vi "Type Conversion.To Double (I8).vi"(3 "value in":i8) -> (1 "value out":dbl)   [LabVIEW 2016, in "VeriStand Data.lvlib"]
doc: "Converts the provided values to double floats, preserving the numerical value of the data."
uses:
  VeriStand Data.lvlib
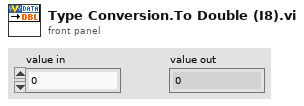
[diagram p1: front panel]
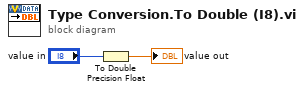
[diagram p0: block diagram]
diagram:
  n1 = To Double Precision Float(number="value in") -> (double precision float=→"value out":dbl)
